vi "findMag.vi"(0 "times":dbl[](array[numeric]), 1 "sens":dbl=0.15, 2 "voltages":dbl[](array[numeric]), 3 "error in (no error)":errorcluster, 4 "freq":dbl=1.367) -> (5 "magfound":dbl, 6 "error out":errorcluster)   [LabVIEW 2016]
panel:
  in  "num":dbl=5.0
  out "npeak":dbl
  out "ppeak":dbl
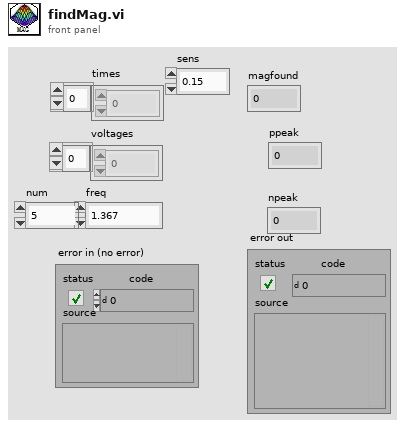
[diagram p1: front panel]
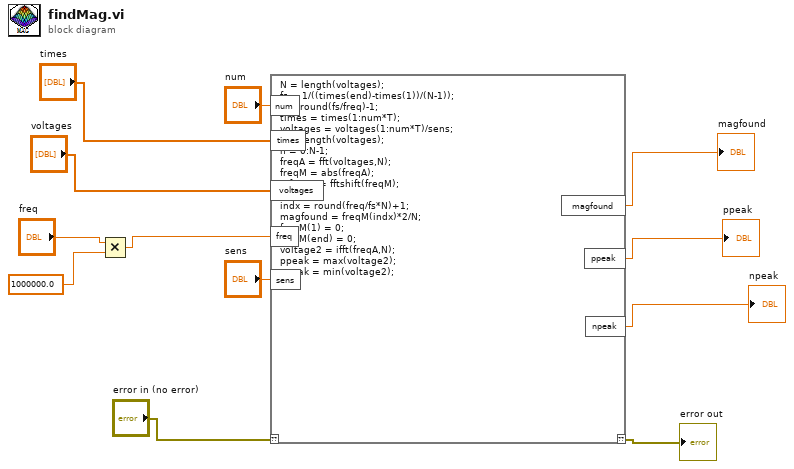
[diagram p0: block diagram]
diagram:
  n1 = Multiply(x="freq", y=1000000.0) -> (x*y=w2:dbl)
  n2 = script code="N = length(voltages);\nfs = 1/((times(end)-times(1))/(N-1));\nT = round(fs/freq)-1;\ntimes = times(1:num*T);\nvoltages = voltages(1:num*T)/sens;\nN = length(voltages);\nn = 0:N-1;\nfreqA = fft(voltages,N);\nfreqM = abs(freqA);\n%freqM = fftshift(freqM);\nf=n*fs/N;\nindx = round(freq/fs*N)+1;\nmagfound = freqM(indx)*2/N;\nfreqM(1) = 0;\nfreqM(end) = 0;\nvoltage2 = ifft(freqA,N);\nppeak = max(voltage2);\nnpeak = min(voltage2);"("??"="error in (no error)", "times"="times", "voltages"="voltages", "freq"=w2, "num"="num", "sens"="sens") -> ("??"=→"error out":errorcluster, "magfound"=→"magfound":dbl, "ppeak"=→"ppeak":dbl, "npeak"=→"npeak":dbl)
